vi "Get Targets and Devices via Storage API.vi"(7 "VI reference (current VI)":refnum<vi>, 8 "error in (no error)":errorcluster, 9 "Main GUID":string="5D441869-002F-93F2-B7E0-78053FA04717", 10 "Tree":refnum<vi>, 11 "NIVS.System Definition Root":refnum<k24>) -> (0 "error out":errorcluster, 3 "NIVS.System Definition Root":refnum<k24>)   [LabVIEW 2019, in "J1939 Workspace Shared.lvlib"]
uses:
  NationalInstruments.VeriStand.SystemStorage
  <vilib>/picture/picture.llb/imagedata.ctl
  J1939 Workspace Shared.lvlib
  NationalInstruments.VeriStand.SystemDefinitionAPI
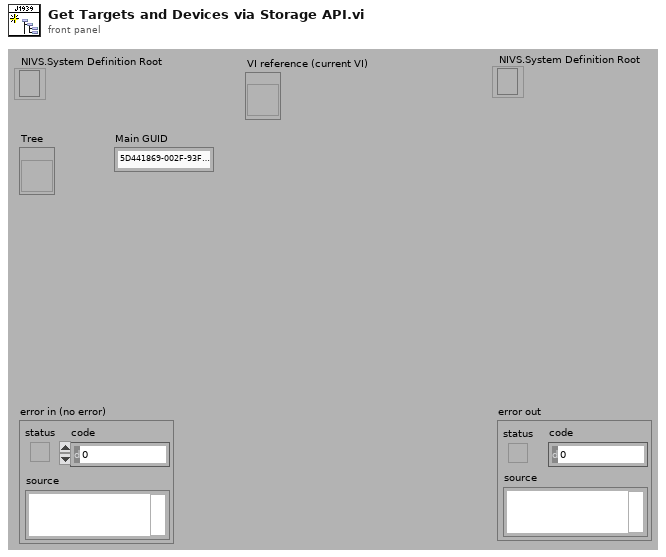
[diagram p1: front panel]
types:
  T1 = typedef "imagedata.ctl" = cluster{"image type":i32, "image depth":i32, "image":u8[], "mask":u8[], "colors":u32[], "Rectangle":cluster{"left":i16, "top":i16, "right":i16, "bottom":i16}}
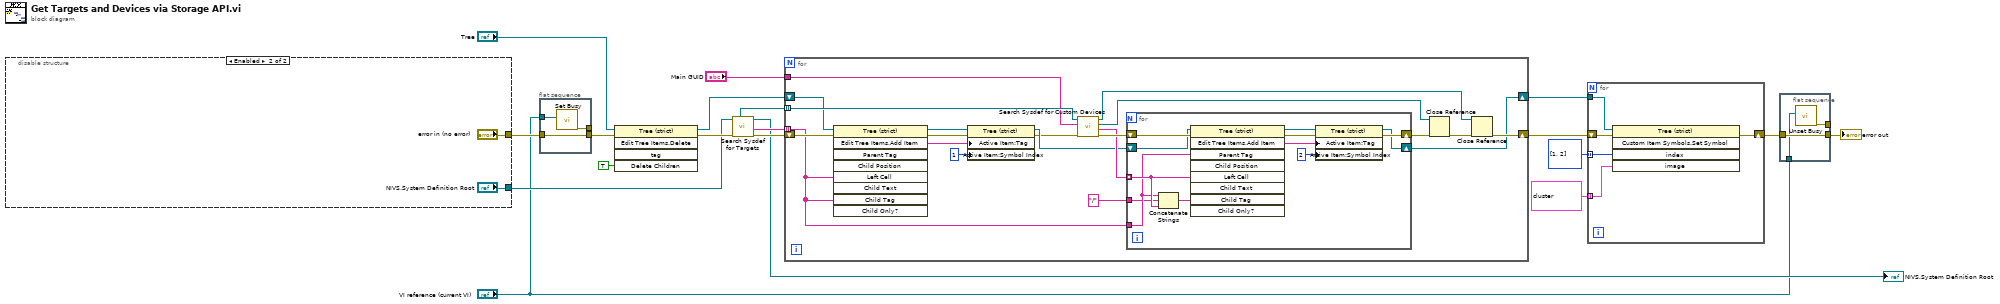
[diagram p0: block diagram]
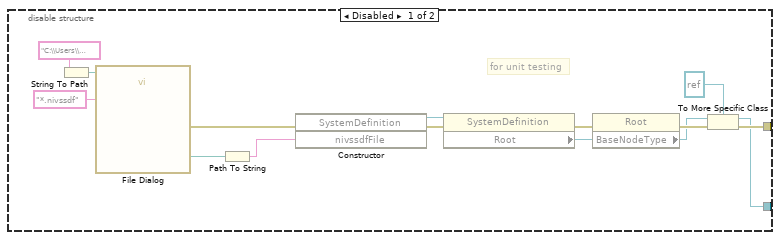
[diagram p2: hidden frame]
diagram:
  n1 = disable-structure shown="Enabled" {
    disable-tunnel: [w21 "NIVS.System Definition Root"] -> w11
    disable-tunnel: [w26 "error in (no error)"] -> w2
    frame Disabled {
      # "for unit testing"
      n2 = String To Path(string="C:\\Users\\Public\\Documents\\National Instruments\\NI VeriStand 2010\\Projects") -> (path=w22:path)
      n3 = call "File Dialog"("start path"=w22, "pattern (all files)"="*.nivssdf") -> ("selected path"=w33:path, "error out"=w20:errorcluster)  [unwired: 10 in, 2 out]
      n4 = Path To String(path=w33) -> (string=w32:string)
      n5 = constructor class="SystemDefinition"(error in=w20, "nivssdfFile"=w32) -> (reference out=w30:refnum<k24>, error out=w31:errorcluster)  [unwired: 2 in, 2 out]
      n6 = property class="SystemDefinition"(reference=w30, error in=w31) -> (error out=w28:errorcluster, "Root"=w29:refnum<k24>)  [unwired: 1 out]
      n7 = property class="Root"(reference=w29, error in=w28) -> (error out=w27:errorcluster, "BaseNodeType"=w25:refnum<k24>)  [unwired: 1 out]
      n8 = To More Specific Class(target class=refnum<k24> refnum, reference=w25, error in=w27) -> (specific class reference=w21:refnum<k24>, error out=w26:errorcluster)
    }
    frame Enabled {
    }
  }
  n9 = flat-sequence {
    tunnel: [w38] -> w17
    tunnel: "VI reference (current VI)" -> [w39]
    tunnel: w2 -> [w38]
    tunnel: [w37] -> _
    frame #0 {
      n10 = call <vilib>:"Set Busy.vi"("VI reference (current VI)"=w39) -> ("error out"=w37:errorcluster)  [unwired: 9 in, 1 out]
    }
  }
  n11 = invoke class="Tree (strict)" method="Edit Tree Items.Delete"(reference="Tree", error in=w17, "Delete Children"=TRUE ("Delete Children?")) -> (reference out=w9:refnum<vi>, error out=w16:errorcluster)  [unwired: 2 in, 3 out]
  n12 = call "Search Sysdef for Targets.vi"("error in (no error)"=w16, "NIVS.System Definition Root"=w11) -> ("error out"=w15:errorcluster, "Target Names"=w19:string[], "NIVS.System Defintion Root Out"=→"NIVS.System Definition Root":refnum<k24>, "Target Nodes"=w14:refnum<k24>[])  [unwired: 6 in]
  n13 = for {
    tunnel: w14 -> [w58] mode=indexing
    tunnel: w19 -> [w50] mode=indexing
    shift-right: [w52] -> w7
    shift-left: w15 -> [w59]
    tunnel: "Main GUID" -> [w48]
    shift-right: [w41] -> w8
    shift-left: w9 -> [w40]
    n14 = invoke class="Tree (strict)" method="Edit Tree Items.Add Item"(reference=w40, error in=w59, "Left Cell"=w50, "Child Tag"=w50) -> (reference out=w46:refnum<vi>, error out=w43:errorcluster, "Edit Tree Items:Add Item"=w44:string)  [unwired: 5 in, 6 out]
    n15 = property class="Tree (strict)"(reference=w46, error in=w43, "Active Item:Tag"=w44, "Active Item:Symbol Index"=1) -> (reference out=w45:refnum<vi>, error out=w42:errorcluster)
    n16 = call "Search Sysdef for Custom Devices.vi"("error in (no error)"=w42, "CD GUID"=w48, "Target Node"=w58) -> ("error out"=w57:errorcluster, "Custom Device Names"=w56:string[], "Custom Device Nodes"=w54:refnum<k24>[], "Target Node Out"=w51:refnum<k24>)  [unwired: 5 in]
    n17 = for {
      tunnel: w56 -> [w70] mode=indexing
      tunnel: w50 -> [w67]
      shift-right: [w61] -> w55
      shift-left: w57 -> [w71]
      tunnel: "/" ("string") -> [w66]
      shift-right: [w60] -> w41
      shift-left: w45 -> [w68]
      n18 = Concatenate Strings(w67, w66, w70) -> (w69:string)
      n19 = invoke class="Tree (strict)" method="Edit Tree Items.Add Item"(reference=w68, error in=w71, "Parent Tag"=w67, "Left Cell"=w70, "Child Tag"=w69) -> (reference out=w64:refnum<vi>, error out=w62:errorcluster, "Edit Tree Items:Add Item"=w63:string)  [unwired: 4 in, 6 out]
      n20 = property class="Tree (strict)"(reference=w64, error in=w62, "Active Item:Tag"=w63, "Active Item:Symbol Index"=2) -> (reference out=w60:refnum<vi>, error out=w61:errorcluster)
    }
    n21 = Close Reference(reference=w54, error in (no error)=w55) -> (error out=w53:errorcluster)
    n22 = Close Reference(reference=w51, error in (no error)=w53) -> (error out=w52:errorcluster)
  }
  n23 = for {
    tunnel: w8 -> [w76]
    shift-right: [w75] -> w5
    shift-left: w7 -> [w73]
    tunnel: i32[] [1, 2] -> [w74] mode=indexing
    tunnel: T1[] [{"image type"=0, "image depth"=32, "image"=array[1024 elements], "mask"=[0, 0, 0, 0, 0, 0, 63, 254, 127, 254, 255, 254, 255, 255, 255, 255, 255, 255, 255, 255, 255, 255, 255, 255, 127, 254, 64, 32, 0, 0, 0, 0], "colors"=[], "Rectangle"={"left"=0, "top"=0, "right"=16, "bottom"=16}}, {"image type"=0, "image depth"=32, "image"=[0, 255, 255, 255, 0, 255, 255, 255, 0, 255, 255, 255, 0, 255, 255, 255, 255, 193, 195, 197, 255, 117, 142, 217, 255, 117, 142, 217, 255, 193, 195, 197, 0, 255, 255, 255, 0, 255, 255, 255, 0, 255, 255, 255, 0, 255, 255, 255, 0, 255, 255, 255, 0, 255, 255, 255, 255, 198, 198, 198, 255, 117, 142, 217, 255, 117, 142, 217, 255, 173, 188, 233, 255, 251, 251, 254, 255, 117, 142, 217, 255, 117, 142, 217, 255, 193, 195, 197, 0, 255, 255, 255, 0, 255, 255, 255, 255, 198, 198, 198, 255, 117, 142, 217, 255, 117, 142, 217, 255, 108, 153, 254, 0, 255, 255, 255, 255, 152, 171, 227, 255, 220, 227, 245, 0, 255, 255, 255, 0, 255, 255, 255, 0, 255, 255, 255, 255, 117, 142, 217, 255, 191, 194, 197, 255, 38, 82, 217, 255, 102, 152, 254, 0, 255, 255, 255, 0, 255, 255, 255, 0, 255, 255, 255, 255, 186, 198, 236, 255, 186, 198, 236, 0, 255, 255, 255, 0, 255, 255, 255, 0, 255, 255, 255, 255, 82, 145, 252, 255, 18, 18, 118, 255, 25, 82, 255, 255, 61, 84, 234, 255, 116, 137, 243, 0, 255, 255, 255, 0, 255, 255, 255, 255, 156, 174, 228, 255, 152, 171, 227, 0, 255, 255, 255, 255, 95, 145, 252, 255, 11, 12, 132, 255, 12, 12, 133, 255, 1, 1, 127, 255, 25, 82, 255, 0, 255, 255, 255, 255, 25, 82, 255, 255, 50, 81, 238, 255, 50, 81, 238, 255, 133, 155, 222, 255, 139, 160, 223, 255, 11, 12, 133, 255, 12, 13, 133, 255, 1, 1, 126, 0, 255, 255, 255, 255, 9, 9, 105, 255, 25, 82, 255, 0, 255, 255, 255, 0, 255, 255, 255, 0, 255, 255, 255, 255, 50, 81, 238, 255, 50, 81, 238, 255, 11, 12, 133, 255, 12, 13, 133, 0, 255, 255, 255, 0, 255, 255, 255, 0, 255, 255, 255, 255, 9, 9, 103, 255, 25, 82, 255, 0, 255, 255, 255, 0, 255, 255, 255, 255, 225, 230, 246, 255, 173, 188, 233, 255, 50, 81, 238, 255, 11, 12, 133, 255, 170, 185, 230, 255, 218, 223, 239, 0, 255, 255, 255, 0, 255, 255, 255, 255, 10, 10, 102, 255, 25, 82, 255, 0, 255, 255, 255, 255, 182, 195, 235, 255, 147, 167, 226, 255, 233, 237, 249, 255, 50, 81, 238, 255, 11, 12, 132, 255, 228, 232, 244, 255, 143, 163, 221, 255, 175, 188, 227, 0, 255, 255, 255, 255, 11, 11, 102, 255, 25, 82, 255, 255, 156, 174, 228, 255, 190, 202, 237, 0, 255, 255, 255, 0, 255, 255, 255, 255, 50, 81, 237, 255, 11, 12, 131, 0, 255, 255, 255, 0, 255, 255, 255, 255, 181, 193, 227, 255, 149, 167, 220, 255, 11, 11, 101, 255, 48, 92, 227, 255, 33, 81, 249, 0, 255, 255, 255, 0, 255, 255, 255, 0, 255, 255, 255, 255, 48, 76, 235, 255, 1, 1, 127, 0, 255, 255, 255, 0, 255, 255, 255, 0, 255, 255, 255, 255, 13, 13, 125, 255, 35, 36, 101, 255, 190, 193, 197, 255, 37, 82, 217, 255, 37, 82, 217, 0, 255, 255, 255, 0, 255, 255, 255, 255, 48, 77, 234, 255, 1, 1, 126, 0, 255, 255, 255, 0, 255, 255, 255, 255, 35, 36, 103, 255, 35, 36, 103, 255, 171, 176, 184, 0, 255, 255, 255, 0, 255, 255, 255, 255, 186, 190, 196, 255, 49, 82, 178, 255, 48, 81, 177, 255, 58, 79, 228, 255, 12, 12, 130, 255, 35, 36, 105, 255, 34, 35, 102, 255, 172, 177, 185, 0, 255, 255, 255, 0, 255, 255, 255, 0, 255, 255, 255, 0, 255, 255, 255, 0, 255, 255, 255, 0, 255, 255, 255, 255, 191, 193, 195, 255, 49, 81, 175, 255, 35, 36, 105, 255, 175, 181, 189, 0, 255, 255, 255, 0, 255, 255, 255, 0, 255, 255, 255, 0, 255, 255, 255], "mask"=[15, 0, 63, 192, 246, 48, 198, 48, 230, 240, 191, 208, 143, 16, 159, 144, 191, 208, 230, 112, 198, 48, 230, 112, 63, 192, 15, 0], "colors"=[], "Rectangle"={"left"=0, "top"=0, "right"=12, "bottom"=14}}] ("Array") -> [w72] mode=indexing
    n24 = invoke on="Invoke Node" class="Tree (strict)" method="Custom Item Symbols.Set Symbol"(reference=w76, error in=w73, "index"=w74, "image"=w72) -> (error out=w75:errorcluster)  [unwired: 1 in, 4 out]
  }
  n25 = flat-sequence {
    tunnel: w5 -> [w79]
    tunnel: [w79] -> w12
    tunnel: [w78] -> _
    tunnel: "VI reference (current VI)" -> [w77]
    frame #0 {
      n26 = call <vilib>:"Unset Busy.vi"("VI reference (current VI)"=w77) -> ("error out"=w78:errorcluster)  [unwired: 10 in]
    }
  }
  "error out" <- w12
